vi "testing search for sequence.vi"(4 "Test Station? (f)":bool, 6 "User":T3, 7 "Header In":string, 8 "error in (no error)":errorcluster, 9 "TestSeqId (\"\")":string, 10 "Action (\"Search\")":string="Search", 11 "Connection Refnum":T1) -> (0 "error out":errorcluster, 1 "Template Keys":T2, 2 "Template":string, 3 "Connection Refnum":T1, 5 "new Header":string)   [LabVIEW 2011]
uses:
  server/database/Users/User Record.ctl
  ITK EXT/utils/keyedarr.llb/Keyed Array.ctl
  Summitek EXT/ODBC/SQL Controls/Connection Refnum.ctl
  ITK EXT/utils/strutil.llb/Case Matching.ctl
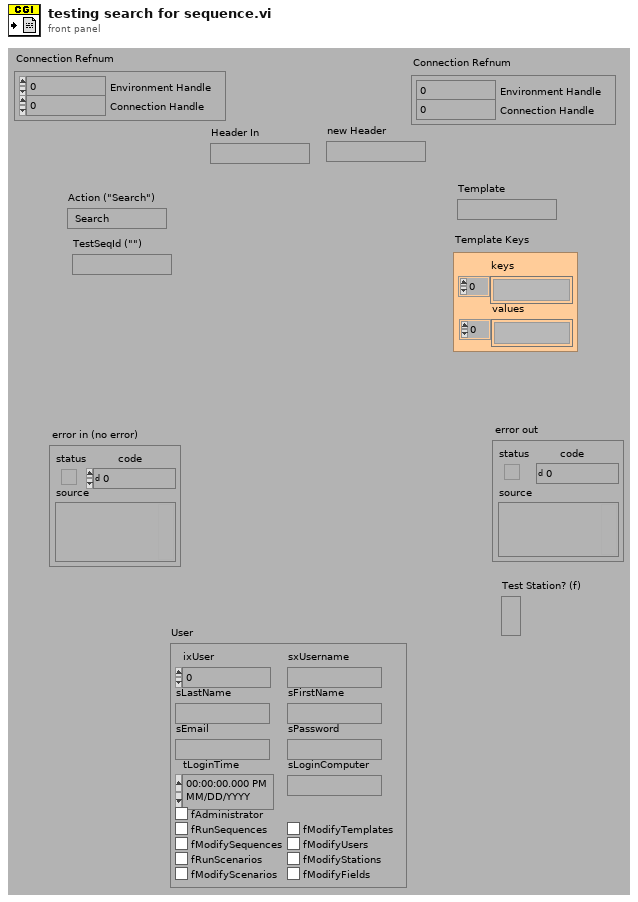
[diagram p1: front panel]
types:
  T1 = typedef "Connection Refnum.ctl" = cluster{"Environment Handle":i32, "Connection Handle":i32}
  T2 = typedef "Keyed Array.ctl" = cluster{"keys":string[], "values":string[]}
  T3 = typedef "User Record.ctl" = cluster{"ixUser":i32, "sxUsername":string, "sLastName":string, "sFirstName":string, "sEmail":string, "sPassword":string, "tLoginTime":timestamp, "sLoginComputer":string, "fAdministrator":bool, "fRunSequences":bool, "fModifySequences":bool, "fRunScenarios":bool, "fModifyScenarios":bool, "fModifyTemplates":bool, "fModifyUsers":bool, "fModifyStations":bool, "fModifyFields":bool}
  T4 = typedef "Sequence Record.ctl" = cluster{"ixSequence":i32, "sxSequenceId":string, "sDescription":string, "sCreator":string, "tCreationDate":timestamp, "sModifier":string, "tModifiedDate":timestamp, "fApproved":bool, "fSpartanSetsSN":bool, "fOverwriteData":bool, "fStopOnFail":bool, "fDisableQuickMode":bool, "fPartialExecution":bool, "fAutoNextItem":bool, "fDoNotPrintOnFail":bool}
  T5 = typedef "Case Matching.ctl" = enum16{"a != A", "a == A", "system"}
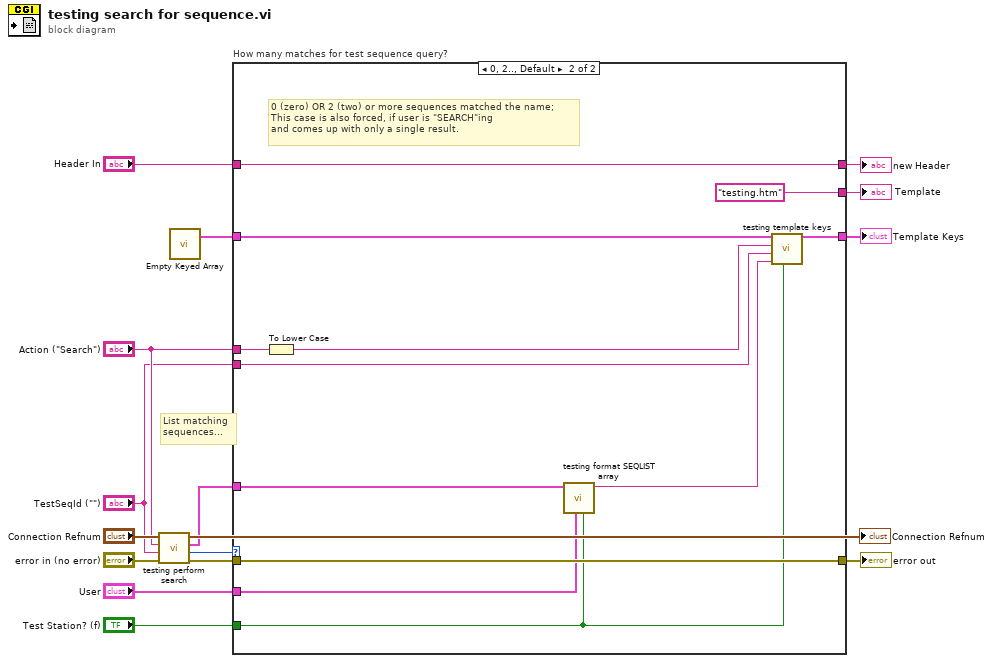
[diagram p0: block diagram]
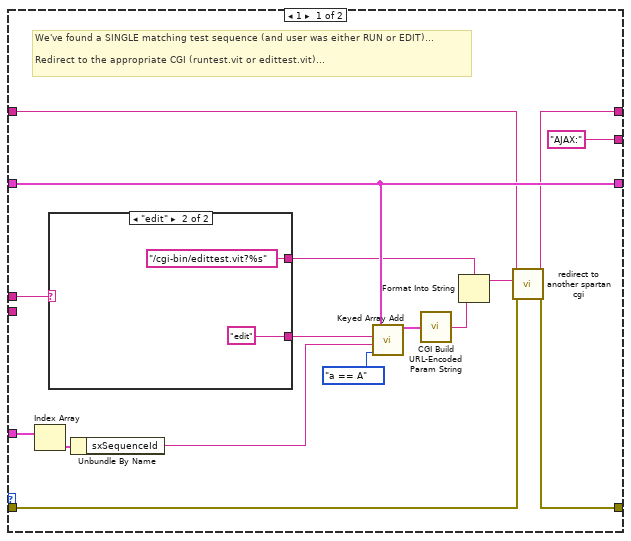
[diagram p2: hidden frame]
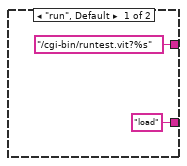
[diagram p3: hidden frame]
diagram:
  # "List matching\nsequences..."
  n1 = call "testing perform search.vi"("error in (no error)"="error in (no error)", "TestSeqId (\"\")"="TestSeqId (\"\")", "Action (\"Search\")"="Action (\"Search\")", "Connection Refnum"="Connection Refnum") -> ("error out"=w3:errorcluster, "Matching Results"=w4:i32, "Results"=w5:T4[], "Connection Refnum"=→"Connection Refnum":T1)  [unwired: 1 in, 3 out]
  n2 = call "Empty Keyed Array.vi"() -> ("empty keyed array"=w13:T2)  [unwired: 3 out]
  n3 = case "How many matches for test sequence query?" shown="0, 2.., Default" w4 {
    tunnel: "TestSeqId (\"\")" -> [_ w40]
    tunnel: w5 -> [w28 w45]
    tunnel: "User" -> [_ w37]
    tunnel: [w29 w43] -> w16
    tunnel: w13 -> [w29 w39]
    tunnel: w3 -> [w31 w48]
    tunnel: [w32 w48] -> w15
    tunnel: ["AJAX:" "testing.htm" ("key")] -> w14
    tunnel: "Action (\"Search\")" -> [w18 w47]
    tunnel: [w25 w46] -> w11
    tunnel: "Header In" -> [w26 w46]
    tunnel: "Test Station? (f)" -> [_ w38]
    frame 1 {
      # "We've found a SINGLE matching test sequence (and user was either RUN or EDIT)...\n\nRedirect to the appropriate CGI (runtest.vit or edittest.vit)..."
      n4 = Index Array(array=w28) -> (element=w30:T4)  [unwired: 1 in]
      n5 = case shown="\"edit\"" w18 {
        tunnel: ["load" ("key") "edit" ("key")] -> w19
        tunnel: ["/cgi-bin/runtest.vit?%s" ("New URL (/cgi-bin/testing.vit)") "/cgi-bin/edittest.vit?%s" ("New URL (/cgi-bin/testing.vit)")] -> w17
        frame "run", Default {
        }
        frame "edit" {
        }
      }
      n6 = Unbundle By Name(w30) -> ("sxSequenceId"=w20:string)
      n7 = call "Keyed Array Add.vi"("case matching (sensitive)"=Case_Matching."a == A", "value"=w20, "key"=w19, "array in"=w29) -> ("array out"=w23:T2)  [unwired: 3 out]
      n8 = call "CGI Build URL-Encoded Param String.vi"("params"=w23) -> ("url-encoded param string"=w22:string)
      n9 = Format Into String(format string=w17, w22) -> (resulting string=w21:string)  [unwired: 2 in, 1 out]
      n10 = call "redirect to another spartan cgi.vi"("error in (no error)"=w31, "New URL (/cgi-bin/testing.vit)"=w21, "Original Header In (to be replaced)"=w26) -> ("error out"=w32:errorcluster, "Redirection Header"=w25:string)  [unwired: 1 in, 6 out]
    }
    frame 0, 2.., Default {
      # "0 (zero) OR 2 (two) or more sequences matched the name;\nThis case is also forced, if user is \"SEARCH\"ing\nand comes up with only a single result."
      n11 = To Lower Case(string=w47) -> (all lower case string=w42:string)
      n12 = call "testing format SEQLIST array.vi"("Test Station? (f)"=w38, "User Information"=w37, "Results"=w45) -> ("SEQLIST array"=w41:string)  [unwired: 8 out]
      n13 = call "testing template keys.vi"("Test Station? (f)"=w38, "$$SEQLIST$$ (\"\")"=w41, "$$SEQID$$ (\"\")"=w40, "$$MODE$$ (\"\")"=w42, "Keys In"=w39) -> ("Keys Out"=w43:T2)  [unwired: 1 in, 5 out]
    }
  }
  "error out" <- w15
  "Template Keys" <- w16
  "Template" <- w14
  "new Header" <- w11
